vi "goto_pos.vi"(6 "Speed (um/s)":i32, 8 "error in (no error)":errorcluster, 9 "New position (nm)":i32[](array[numeric]), 10 "device ID":i32, 11 "Handle in":i64) -> (0 "error out":errorcluster, 2 "Return (<0 is error)":i32, 3 "Handle out":i64)   [LabVIEW 2016, in "OSB_uMp_library.lvlib"]
doc: "Sends uMp to a specified location (location coordinates in nm).\n\nNew position (nm) should be an array with three elements, representing x, y, and z values.\nVI returns custom error code -8005 on the LabVIEW error cluster if the array is of the wrong length."
uses:
  OSB_uMp_library.lvlib
  ump.dll
panel:
  # "By Stuart Box at OxSyBio Ltd, 2017\n\nThis software is provided WITHOUT ANY WARRANTY; without even the implied warranty of MERCHANTABILITY or FITNESS FOR A PARTICULAR PURPOSE.\n\ninfo@oxsybio.com\n\nOxSyBio Ltd, The Walbrook Building, 25 Walbrook, London, EC4N 8AF"
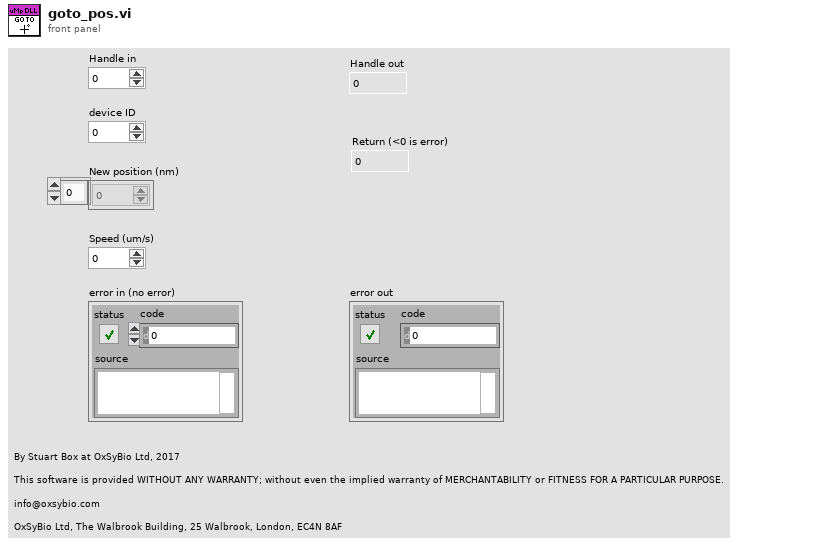
[diagram p1: front panel]
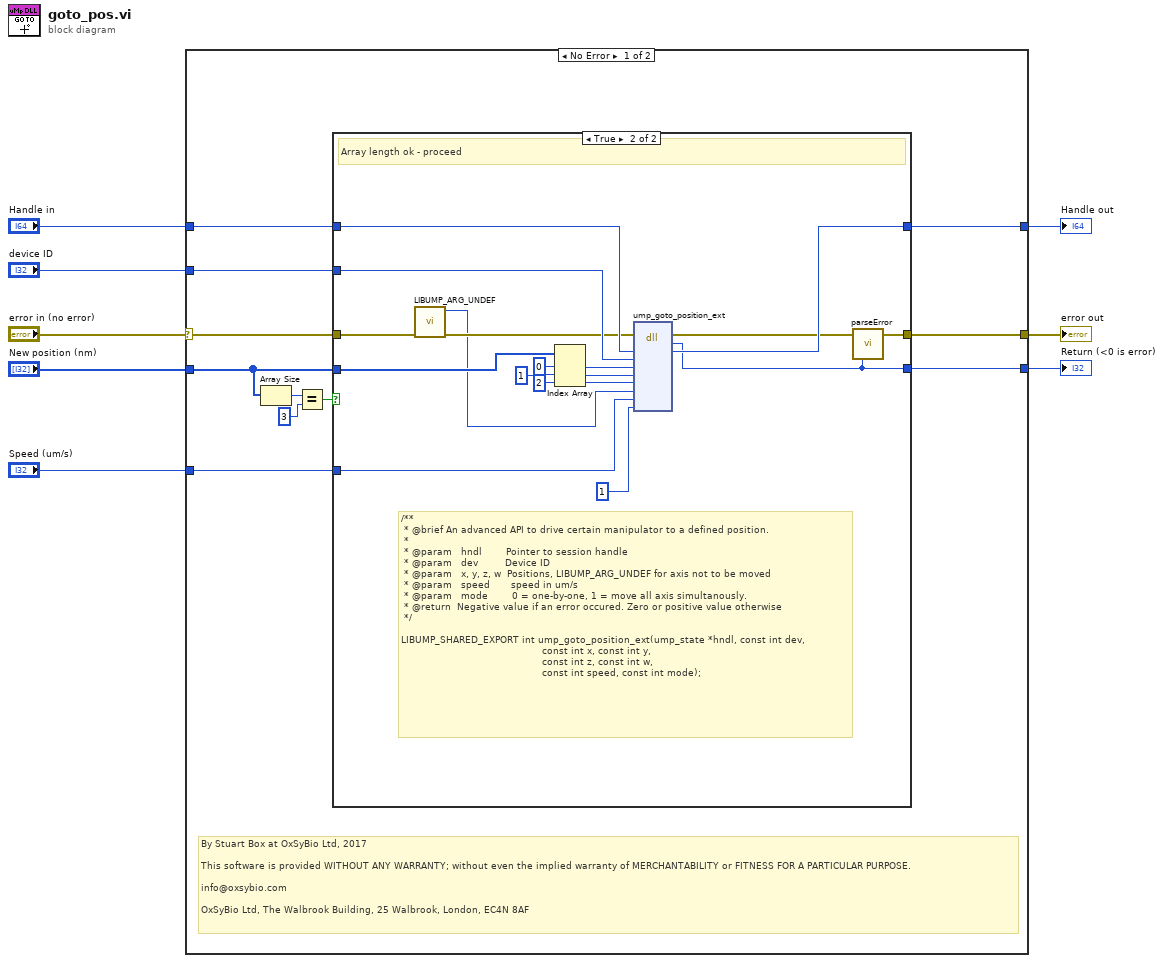
[diagram p0: block diagram]
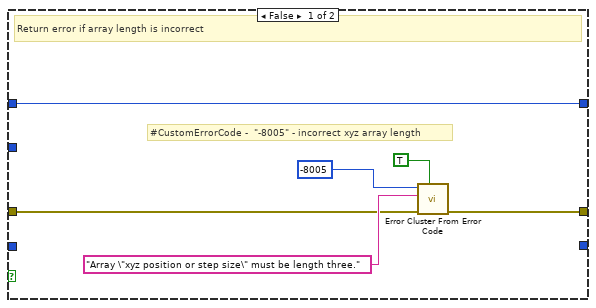
[diagram p2: hidden frame]
diagram:
  n1 = case shown="No Error" "error in (no error)" {
    selector: "error in (no error)" -> [w9 w45]
    tunnel: "Speed (um/s)" -> [w19 _]
    tunnel: "device ID" -> [w18 _]
    tunnel: "Handle in" -> [w17 w44]
    tunnel: [w16 _] -> w5
    tunnel: [w15 w45] -> w4
    tunnel: [w14 w44] -> w3
    tunnel: "New position (nm)" -> [w11 _]
    frame No Error {
      # "By Stuart Box at OxSyBio Ltd, 2017\n\nThis software is provided WITHOUT ANY WARRANTY; without even the implied warranty of MERCHANTABILITY or FITNESS FOR A PARTICULAR PURPOSE.\n\ninfo@oxsybio.com\n\nOxSyBio Ltd, The Walbrook Building, 25 Walbrook, London, EC4N 8AF"
      n2 = Array Size(array=w11) -> (size(s)=w12:i32)
      n3 = Equal?(x=w12, y=3) -> (x = y?=w10:bool)
      n4 = case shown="True" w10 {
        tunnel: w11 -> [_ w43]
        tunnel: w19 -> [_ w38]
        tunnel: w18 -> [_ w37]
        tunnel: w17 -> [w25 w36]
        tunnel: [_ w26] -> w16
        tunnel: [w20 w27] -> w15
        tunnel: [w25 w35] -> w14
        tunnel: w9 -> [w21 w30]
        frame False {
          # "#CustomErrorCode -  \"-8005\" - incorrect xyz array length"
          # "Return error if array length is incorrect"
          n5 = call <vilib>:"Error Cluster From Error Code.vi"("show call chain? (False)"=TRUE, "error in (no error)"=w21, "error message (\"\")"="Array \"xyz position or step size\" must be length three." ("error message (\"\")"), "error code (0)"=-8005) -> ("error out"=w20:errorcluster)  [unwired: 5 in]
        }
        frame True {
          # "/**\n * @brief An advanced API to drive certain manipulator to a defined position.\n *\n * @param   hndl        Pointer to session handle\n * @param   dev         Device ID\n * @param   x, y, z, w  Positions, LIBUMP_ARG_UNDEF for axis not to be moved\n * @param   speed       speed in um/s\n * @param   mode        0 = one-by-one, 1 = move all axis simultanously.\n * @return  Negative value if an error occured. Zero or positive value otherwise\n */\n\nLIBUMP_SHARED_EXPORT int ump_goto_position_ext(ump_state *hndl, const int dev,\n                                               const int x, const int y,\n                                               const int z, const int w,\n                                               const int speed, const int mode);"
          # "Array length ok - proceed"
          n6 = call "LIBUMP_ARG_UNDEF.vi"("Error In"=w30) -> ("Error Out"=w31:errorcluster, "LIBUMP_ARG_UNDEF"=w29:i32)  [unwired: 9 in]
          n7 = Index Array(array=w43, index #1=0 ("index"), index #2=1 ("index"), index #3=2 ("index")) -> (element #1=w34:i32, element #2=w33:i32, element #3=w32:i32)
          n8 = dll-call lib="C:/Users/Stu/Desktop/OSB LabVIEW uMp/uMp_library/ump.dll" fn="ump_goto_position_ext"(error in=w31, "handle"=w36, "dev"=w37, "x"=w34, "y"=w33, "z"=w32, "w"=w29, "speed"=w38, "mode"=1) -> (error out=w28:errorcluster, "return"=w26:i32, "handle"=w35:i64)  [unwired: 9 in, 1 out]
          n9 = call "parseError.vi"("Error In"=w28, "ump dll return value (<0 is error)"=w26) -> ("Error Out"=w27:errorcluster)  [unwired: 24 in, 1 out]
        }
      }
    }
    frame Error {
    }
  }
  "Return (<0 is error)" <- w5
  "error out" <- w4
  "Handle out" <- w3
